vi "SlideFIFO.vi"(2 "shift (photons)":u32, 3 "window (photons)":u32, 4 "rawdata":T1) -> (0 "SlideTime":dbl[](array[numeric]) format="%.2f", 1 "SlideMCS":u32[][](array[numeric]))   [LabVIEW 2009]
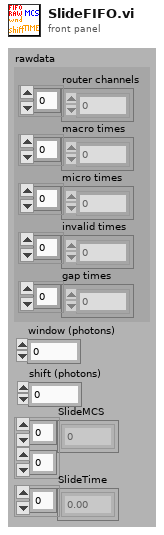
[diagram p1: front panel]
types:
  T1 = cluster{"router channels":u8[], "macro times":u32[], "micro times":u16[], "invalid times":u32[], "gap times":u32[]}
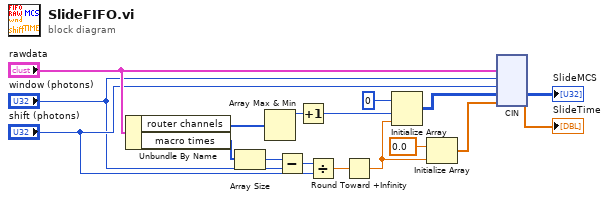
[diagram p0: block diagram]
diagram:
  n1 = Unbundle By Name("rawdata") -> ("router channels"=w15:u8[], "macro times"=w12:u32[])
  n2 = Array Size(array=w12) -> (size(s)=w11:i32)
  n3 = Array Max & Min(array=w15) -> (max value=w14:u8)  [unwired: 3 out]
  n4 = Subtract(x=w11, y="window (photons)") -> (x-y=w10:u32)
  n5 = Increment(x=w14) -> (x+1=w13:u8)
  n6 = Divide(x=w10, y="shift (photons)") -> (x/y=w8:dbl)
  n7 = Round Toward +Infinity(x=w8) -> (ceil(x): smallest int >= x=w5:dbl)
  n8 = Initialize Array(u32 0 ("element"), w13, w5) -> (w2:u32[][])
  n9 = Initialize Array(0.0 ("element"), w5) -> (w4:dbl[])
  n10 = cin("rawdata", "window (photons)", "shift (photons)", w2, w4) -> (→"SlideMCS":u32[][], →"SlideTime":dbl[])  [unwired: 3 in]
